vi "BackpackController.vi"(10 "Joystick":bool[](array[boolean]), 11 "SolenoidDevRef":T1={"DevStatus"={"status"=FALSE, "code"=0, "source"=""}, "Pneumatics Control Module"=0, "Forward Solenoid Channel"=enum."Invalid", "Reverse Solenoid Channel"=enum."Invalid"}) -> ()   [LabVIEW 2014]
uses:
  <vilib>/Rock Robotics/WPI/Solenoid/WPI_SolenoidDevRef.ctl
  <vilib>/Rock Robotics/WPI/Solenoid/WPI_SolenoidChannel.ctl
  <vilib>/Rock Robotics/WPI/Solenoid/WPI_SolenoidValue.ctl
  <vilib>/Rock Robotics/WPI/Solenoid/WPI_SolenoidSetEnum.vi
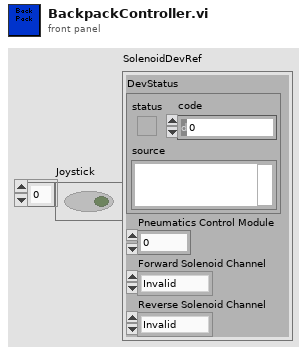
[diagram p1: front panel]
types:
  T1 = typedef "WPI_SolenoidDevRef.ctl" = cluster{"DevStatus":errorcluster, "Pneumatics Control Module":u8, "Forward Solenoid Channel":T2, "Reverse Solenoid Channel":T2}
  T2 = typedef "WPI_SolenoidChannel.ctl" = enum8{"Solenoid 0", "Solenoid 1", "Solenoid 2", "Solenoid 3", "Solenoid 4", "Solenoid 5", "Solenoid 6", "Solenoid 7", "Invalid"}
  T3 = typedef "WPI_SolenoidValue.ctl" = enum16{"Off", "On", "Forward", "Reverse"}
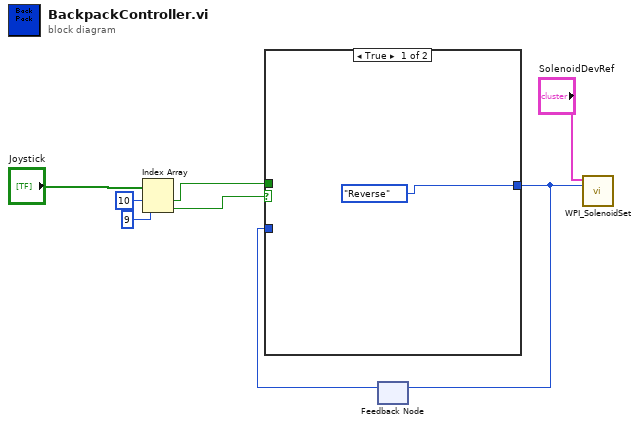
[diagram p0: block diagram]
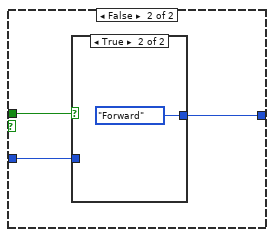
[diagram p2: hidden frame]
diagram:
  n1 = Index Array(array="Joystick", index #1=10 ("index"), index #2=9 ("index")) -> (element #1=w2:bool, element #2=w1:bool)
  n2 = feedback #1() -> (w6:T3)  [unwired: 1 in]
  n3 = case shown="True" w1 {
    tunnel: [WPI_SolenoidValue."Reverse" ("Value") w12] -> w7
    tunnel: w6 -> [_ w11]
    tunnel: w2 -> [_ w10]
    frame True {
    }
    frame False {
      n4 = case shown="True" w10 {
        tunnel: [w13 WPI_SolenoidValue."Forward" ("Value")] -> w12
        tunnel: w11 -> [w13 _]
        frame False {
        }
        frame True {
        }
      }
    }
  }
  n5 = feedback-in #1(w7) -> ()
  n6 = call-poly <vilib>:"WPI_SolenoidSet.vi"("Value"=w7, "SolenoidDevRef"="SolenoidDevRef") -> ()  [unwired: 8 in, 2 out]
